vi "Initialize.vi"(7 "Serial Configuration":T1={"Baud Rate"=57600, "Parity"=1, "Data Bits"=7, "Stop Bits"=10, "Flow Control"=0} {"Flow Control" items=["None", "XON/XOFF", "RTS/CTS", "XON/XOFF & RTS/CTS", "DTR/DSR", "XON/XOFF & DTR/DSR"]; "Stop Bits" items=["1.0"=10, "1.5"=15, "2.0"=20]; "Data Bits" items=["7"=7, "8"=8]; "Parity" items=["None", "Odd", "Even", "Mark", "Space"]; "Baud Rate" items=["300"=300, "600"=600, "1200"=1200, "2400"=2400, "4800"=4800, "9600"=9600, "19200"=19200, "38400"=38400, "57600"=57600]}, 8 "error in (no error)":errorcluster, 9 "Reset (True)":bool=TRUE, 10 "ID Query (True)":bool=TRUE) -> (0 "error out":errorcluster, 3 "VISA resource name out":refnum<visa-resource-name>)   [LabVIEW 2016, in "Lake Shore 350.lvlib"]
doc: "Establishes communication with the instrument and optionally performs an instrument identification query and/or an instrument reset. It also places the instrument in a default state needed for other instrument driver operations. Therefore, call this VI before calling other instrument driver VIs for this instrument. Generally, you need to call the <B>Initialize VI</B> only once at the beginning of an application."
uses:
  Lake Shore 350.lvlib
  Instrument_Setup.vi
panel:
  out "VISA resource name 3":refnum<visa-resource-name>
  # "(c) 2013 Lake Shore Cryotronics Inc.  ALL RIGHTS RESERVED."
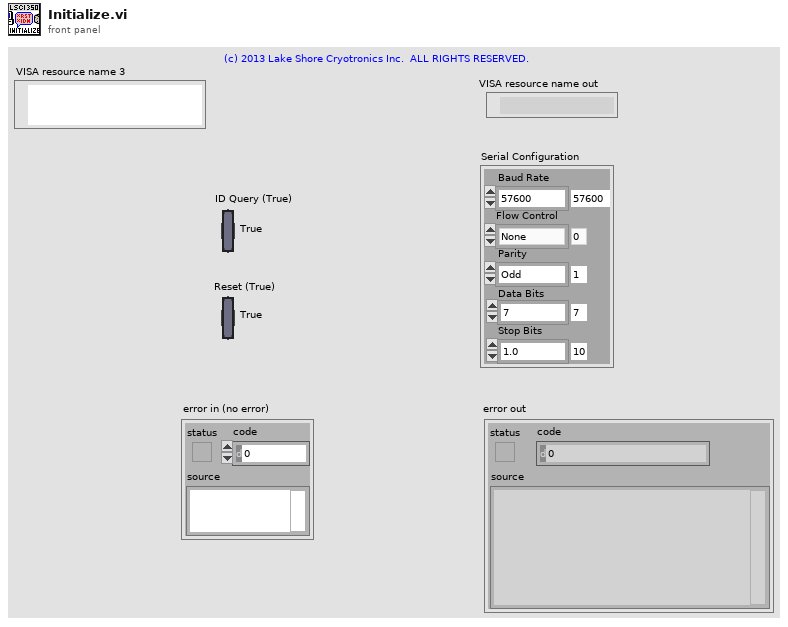
[diagram p1: front panel]
types:
  T1 = cluster{"Baud Rate":u32, "Parity":u16, "Data Bits":u16, "Stop Bits":u16, "Flow Control":u16}
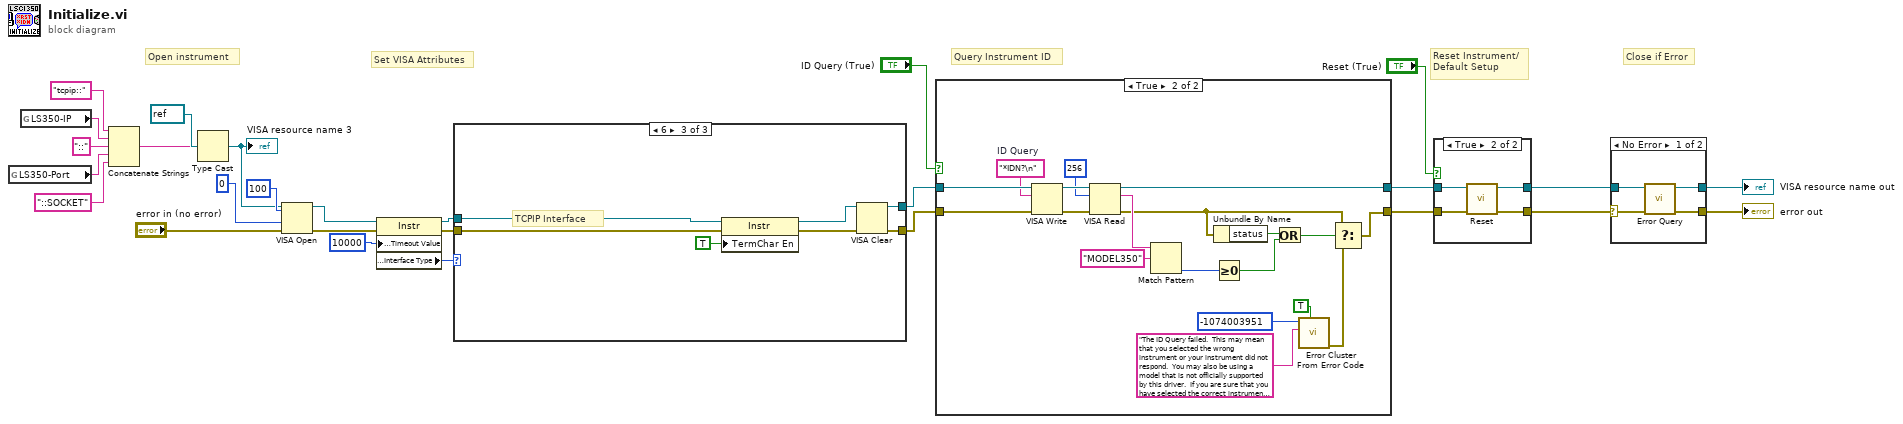
[diagram p0: block diagram]
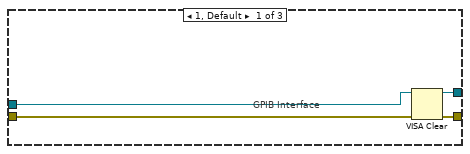
[diagram p2: hidden frame]
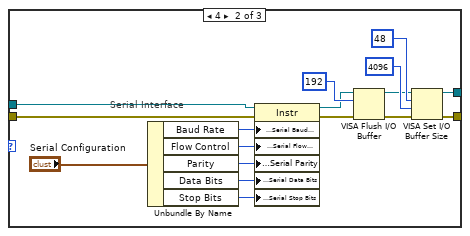
[diagram p3: hidden frame]
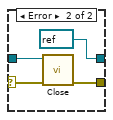
[diagram p4: hidden frame]
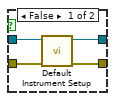
[diagram p5: hidden frame]
diagram:
  # "Set VISA Attributes"
  # "Close if Error"
  # "Query Instrument ID"
  # "Reset Instrument/\nDefault Setup"
  # "Open instrument"
  n1 = global read "Instrument_Setup.vi" "LS350-Port"() -> (w1:string)
  n2 = global read "Instrument_Setup.vi" "LS350-IP"() -> (w2:string)
  n3 = Concatenate Strings("tcpip::" ("string"), w2, "::", w1, "::SOCKET") -> (w9:string)
  n4 = Type Cast(type=refnum<visa-resource-name> refnum ("VISA resource name"), x=w9) -> (*(type *) &x=w5:refnum<visa-resource-name>)
  "VISA resource name 3" <- w5
  n5 = VISA Open(timeout (0)=u32 100 ("VISA Open timeout (0)"), access mode=u32 0, error in (no error)="error in (no error)", VISA resource name=w5) -> (VISA resource name=w17:refnum<visa-resource-name>, error out=w6:errorcluster)  [unwired: 1 in]
  n6 = property class="Instr"(reference=w17, error in=w6, "General Settings:Timeout Value"=u32 10000) -> (reference out=w16:refnum<visa-resource-name>, error out=w15:errorcluster, "Interface Information:Interface Type"=w14:u16)
  n7 = case shown="6" w14 {
    tunnel: [w31 w35 w51] -> w12
    tunnel: [w30 w34 w49] -> w11
    tunnel: w16 -> [w28 w32 w55]
    tunnel: w15 -> [w29 w33 w54]
    frame 1, Default {
      # "GPIB Interface"
      n8 = VISA Clear(VISA resource name=w28, error in (no error)=w29) -> (VISA resource name out=w31:refnum<visa-resource-name>, error out=w30:errorcluster)
    }
    frame 4 {
      # "Serial Interface"
      n9 = Unbundle By Name("Serial Configuration") -> ("Baud Rate"=w43:u32, "Flow Control"=w47:u16, "Parity"=w45:u16, "Data Bits"=w44:u16, "Stop Bits"=w48:u16)
      n10 = property class="Instr"(reference=w32, error in=w33, "Serial Settings:Serial Baud Rate"=w43, "Serial Settings:Serial Flow Control"=w47, "Serial Settings:Serial Parity"=w45, "Serial Settings:Serial Data Bits"=w44, "Serial Settings:Serial Stop Bits"=w48) -> (reference out=w39:refnum<visa-resource-name>, error out=w37:errorcluster)
      n11 = VISA Flush I/O Buffer(VISA resource name=w39, mask (16)=u16 192, error in (no error)=w37) -> (VISA resource name out=w36:refnum<visa-resource-name>, error out=w38:errorcluster)
      n12 = VISA Set I/O Buffer Size(VISA resource name=w36, mask (16)=u16 48, size (4096)=u32 4096 ("size (0)"), error in (no error)=w38) -> (VISA resource name out=w35:refnum<visa-resource-name>, error out=w34:errorcluster)
    }
    frame 6 {
      # "TCPIP Interface"
      n13 = property class="Instr"(reference=w55, error in=w54, "TermChar En"=TRUE) -> (reference out=w52:refnum<visa-resource-name>, error out=w50:errorcluster)
      n14 = VISA Clear(VISA resource name=w52, error in (no error)=w50) -> (VISA resource name out=w51:refnum<visa-resource-name>, error out=w49:errorcluster)
    }
  }
  n15 = case shown="True" "ID Query (True)" {
    tunnel: [w56 w76] -> w26
    tunnel: [w57 w59] -> w27
    tunnel: w12 -> [w57 w74]
    tunnel: w11 -> [w56 w75]
    frame False {
    }
    frame True {
      w60 = "*IDN?\n"  # ID Query
      n16 = VISA Write(VISA resource name=w74, write buffer=w60, error in (no error)=w75) -> (VISA resource name out=w72:refnum<visa-resource-name>, error out=w71:errorcluster)  [unwired: 1 out]
      n17 = VISA Read(VISA resource name=w72, byte count=u32 256, error in (no error)=w71) -> (VISA resource name out=w59:refnum<visa-resource-name>, read buffer=w73:string, error out=w58:errorcluster)  [unwired: 1 out]
      n18 = Match Pattern(string=w73, regular expression="MODEL350") -> (offset past match=w64:i32)  [unwired: 1 in, 3 out]
      n19 = Unbundle By Name(w58) -> ("status"=w63:bool)
      n20 = Greater Or Equal To 0?(x=w64) -> (x >= 0?=w61:bool)
      n21 = Or(x=w63, y=w61) -> (x .or. y?=w62:bool)
      n22 = call <vilib>:"Error Cluster From Error Code.vi"("show call chain? (False)"=TRUE, "error message (\"\")"="The ID Query failed.  This may mean that you selected the wrong instrument or your instrument did not respond.  You may also be using a model that is not officially supported by this driver.  If you are sure that you have selected the correct instrument and it is responding, try disabling the ID Query." ("Source (VI Name)"), "error code (0)"=-1074003951 ("Code")) -> ("error out"=w68:errorcluster)  [unwired: 6 in]
      n23 = Select(t=w58, s=w62, f=w68) -> (s? t:f=w76:errorcluster)
    }
  }
  n24 = case shown="True" "Reset (True)" {
    tunnel: w26 -> [w79 w81]
    tunnel: [w78 w84] -> w20
    tunnel: w27 -> [w80 w82]
    tunnel: [w77 w83] -> w21
    frame False {
      n25 = call "Default Instrument Setup.vi"("error in (no error)"=w79, "VISA resource name"=w80) -> ("error out"=w78:errorcluster, "VISA resource name out"=w77:refnum<visa-resource-name>)  [unwired: 8 in]
    }
    frame True {
      n26 = call "Reset.vi"("error in (no error)"=w81, "VISA resource name"=w82) -> ("error out"=w84:errorcluster, "VISA resource name out"=w83:refnum<visa-resource-name>)  [unwired: 8 in]
    }
  }
  n27 = case shown="No Error" w20 {
    selector: w20 -> [w88 w90]
    tunnel: w21 -> [w87 w91]
    tunnel: [w86 refnum<visa-resource-name> refnum ("VISA resource name out")] -> w23
    tunnel: [w85 w92] -> w22
    frame No Error {
      n28 = call "Error Query.vi"("error in (no error)"=w88, "VISA resource name"=w87) -> ("error out"=w85:errorcluster, "VISA resource name out"=w86:refnum<visa-resource-name>)  [unwired: 7 in, 1 out]
    }
    frame Error {
      n29 = call "Close.vi"("error in (no error)"=w90, "VISA resource name"=w91) -> ("error out"=w92:errorcluster)  [unwired: 9 in]
    }
  }
  "VISA resource name out" <- w23
  "error out" <- w22
